vi "GetNVURLs.vi"(9 "Target Relative":bool, 10 "URL":string, 11 "Owning app":refnum<vi>) -> (2 "Resolved URL":string, 3 "Unresolved URL":string)   [LabVIEW 2017, in "NI_Variable.lvlib"]
uses:
  <vilib>/variable/NI_Variable.lvlib
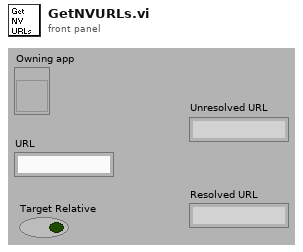
[diagram p1: front panel]
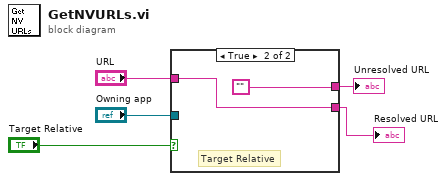
[diagram p0: block diagram]
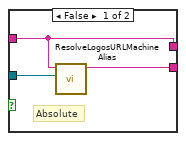
[diagram p2: hidden frame]
diagram:
  n1 = case shown="True" "Target Relative" {
    tunnel: "URL" -> [w7 w10]
    tunnel: [w7 ""] -> w2
    tunnel: [w6 w10] -> w3
    tunnel: "Owning app" -> [w8 _]
    frame False {
      # "Absolute"
      n2 = call <vilib>:"ResolveLogosURLMachineAlias.vi"("App Refnum"=w8, "Unresolved URL"=w7) -> ("Resolved URL"=w6:string)  [unwired: 8 in, 1 out]
    }
    frame True {
      # "Target Relative"
    }
  }
  "Resolved URL" <- w3
  "Unresolved URL" <- w2
